vi "clear Complex Data.vi"(4 "error in (no error)":errorcluster, 7 "Complex Data":refnum<class "Complex Data.lvclass">) -> (0 "error out":errorcluster)   [LabVIEW 2018]
doc: "Destroys a Complex Data object and frees its allocated memory."
uses:
  SpectralRadar/LabVIEW/2012/user.lib/SpectralRadar.llb/Complex Data.lvclass
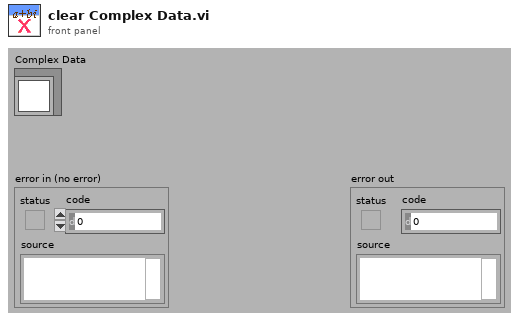
[diagram p1: front panel]
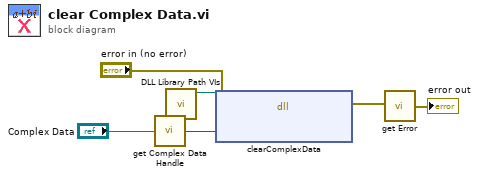
[diagram p0: block diagram]
diagram:
  n1 = call "get Complex Data Handle.vi"("Complex Data"="Complex Data") -> ("Handle"=w5:u64)
  n2 = call "DLL Library Path VIs.vi"() -> ("SpectralRadarDLL"=w1:path)  [unwired: 8 in, 3 out]
  n3 = dll-call lib="C:/Project/SerialSectOCT - FFT GPU/SerialSectOCT/Labview Software/DLL/SpectralRadar.dll" fn="clearComplexData"(path in=w1, error in="error in (no error)", "Complex Data Handle"=w5) -> (error out=w4:errorcluster)  [unwired: 3 in, 1 out]
  n4 = call "get Error.vi"("error in (no error)"=w4) -> ("error out"=→"error out":errorcluster)
